vi "getDTFromXmlNative.vi"(8 "error in (no error)":errorcluster, 10 "eventXML":refnum<k20>, 11 "ScriptEvent in":refnum<class "ScriptEvent.lvclass">) -> (0 "error out":errorcluster, 2 "eventXML out":refnum<k20>, 3 "ScriptEvent out":refnum<class "ScriptEvent.lvclass">)   [LabVIEW 2011, in "Tools.lvlib" / "Scripting.lvlib" / "ScriptEvent.lvclass"]
uses:
  ScriptEvent.lvclass
  ScriptEvent.lvclass/ScriptEvent.ctl
  <vilib>/xml/Close Reference(Node).vi
  <vilib>/xml/NI_XML.lvlib
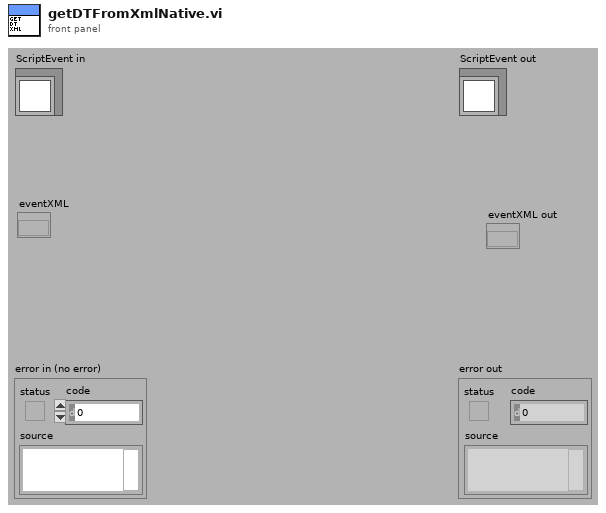
[diagram p1: front panel]
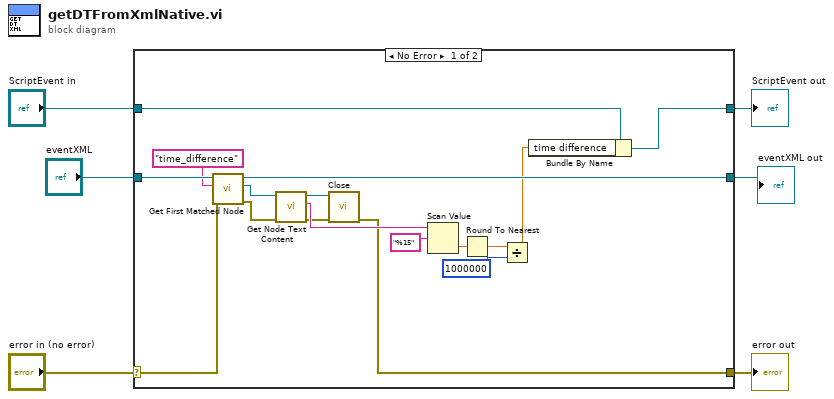
[diagram p0: block diagram]
diagram:
  n1 = case shown="No Error" "error in (no error)" {
    selector: "error in (no error)" -> [w8 w25]
    tunnel: [w9 w25] -> w5
    tunnel: [w10 w24] -> w3
    tunnel: "ScriptEvent in" -> [w11 w24]
    tunnel: "eventXML" -> [w23 _]
    tunnel: [w13 _] -> w1
    frame No Error {
      n2 = call <vilib>:"Get First Matched Node.vi"("error in (no error)"=w8, "XPath expression"="time_difference", "node in"=w23) -> ("error out"=w18:errorcluster, "node result"=w17:refnum<k20>, "node out"=w13:refnum<k20>)  [unwired: 6 in]
      n3 = call <vilib>:"Get Node Text Content.vi"("error in (no error)"=w18, "node in"=w17) -> ("error out"=w15:errorcluster, "node text"=w16:string, "node out"=w14:refnum<k20>)  [unwired: 7 in]
      n4 = call-poly <vilib>:"Close.vi"("error in (no error)"=w15, "node"=w14) -> ("error out"=w9:errorcluster)  [unwired: 7 in]
      n5 = Scan Value(string=w16, format string="%15") -> (value=w19:dbl)  [unwired: 1 in, 1 out]
      n6 = Round To Nearest(number=w19) -> (nearest integer value=w7:dbl)
      n7 = Divide(x=w7, y=1000000) -> (x/y=w12:dbl)
      n8 = Bundle By Name(cluster=w11, "time difference"=w12) -> (w10:refnum<class "ScriptEvent.lvclass">)
    }
    frame Error {
    }
  }
  "error out" <- w5
  "ScriptEvent out" <- w3
  "eventXML out" <- w1
